vi "Change Handler Log Level.vi"(8 "error in":errorcluster, 10 "New Log Level":T1, 11 "Handler Name":string) -> (0 "error out":errorcluster)   [LabVIEW 2024, in "hse-logger.lvlib"]
doc: "Change the log level of the given log-handler.\n\n____\nHAMPEL SOFTWARE ENGINEERING v2.2.2 (2025-01-16 15:41)"
uses:
  <vilib>/Hampel Software Engineering/HSE Logger/hse-logger.lvlib
  <vilib>/Hampel Software Engineering/HSE Logger/LogLevel.ctl
  <vilib>/Hampel Software Engineering/HSE Logger/Logger/Logger.lvclass
  <vilib>/Hampel Software Engineering/HSE Logger/Handler/Handler.lvclass
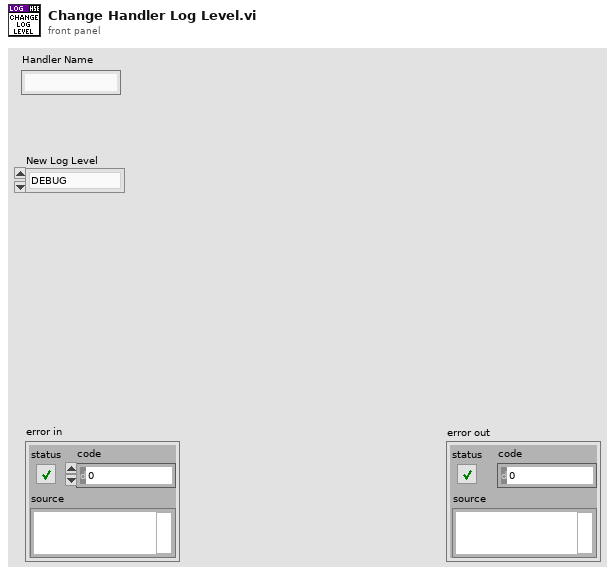
[diagram p1: front panel]
types:
  T1 = typedef "hse-logger.lvlib/LogLevel.ctl" = enum16{"DEBUG", "INFO", "WARNING", "ERROR", "CRITICAL"}
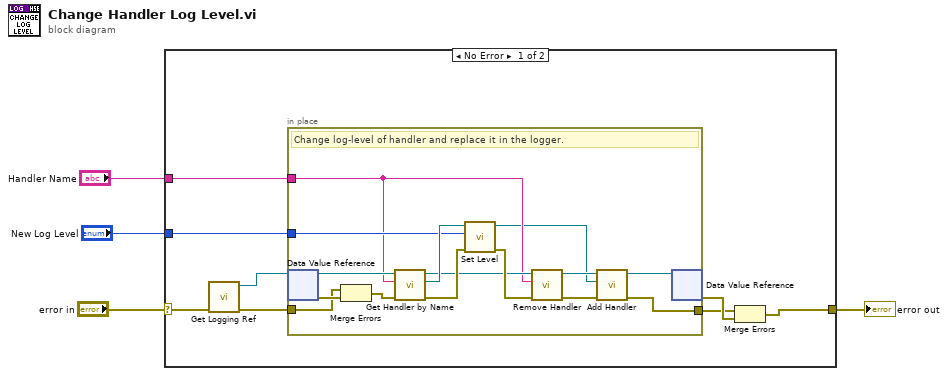
[diagram p0: block diagram]
diagram:
  n1 = case shown="No Error" "error in" {
    selector: "error in" -> [w12 w28]
    tunnel: "Handler Name" -> [w9 _]
    tunnel: "New Log Level" -> [w8 _]
    tunnel: [w5 w28] -> w1
    frame No Error {
      n2 = call <vilib>:"Get Logging Ref.vi"("error in"=w12) -> ("error out"=w7:errorcluster, "Logger DVR"=w11:refnum<data-value>)  [unwired: 9 in]
      n3 = in-place {
        in-place-border: w9 -> [w20]
        in-place-border: w8 -> [w22]
        in-place-border: w7 -> [w14]
        in-place-border: [w13] -> w6
        # "Change log-level of handler and replace it in the logger."
        n4 = in-place-dvr #1(w11) -> (w26:refnum<class "Logger.lvclass">, w25:errorcluster)
        n5 = Merge Errors(w14, w25) -> (w15:errorcluster)
        n6 = call-dynamic "Get Handler by Name.vi"("error in"=w15, "Name"=w20, "Logger in"=w26) -> ("error out"=w24:errorcluster, "Handler out"=w23:refnum<class "Handler.lvclass">, "Logger out"=w21:refnum<class "Logger.lvclass">)  [unwired: 6 in]
        n7 = call-dynamic "Set Level.vi"("error in"=w24, "Level"=w22, "Handler in"=w23) -> ("error out"=w27:errorcluster, "Handler out"=w17:refnum<class "Handler.lvclass">)  [unwired: 7 in]
        n8 = call-dynamic "Remove Handler.vi"("error in"=w27, "Name"=w20, "Logger in"=w21) -> ("error out"=w19:errorcluster, "Logger out"=w18:refnum<class "Logger.lvclass">)  [unwired: 7 in]
        n9 = call <vilib>:"Add Handler.vi"("error in"=w19, "Handler"=w17, "Logger in"=w18) -> ("error out"=w13:errorcluster, "Logger out"=w16:refnum<class "Logger.lvclass">)  [unwired: 7 in]
        n10 = in-place-dvr #1(w16) -> (w10:errorcluster)  [unwired: 1 out]
      }
      n11 = Merge Errors(w6, w10) -> (w5:errorcluster)
    }
    frame Error {
    }
  }
  "error out" <- w1
